vi "Release Session.vi"(8 "error in (no error)":errorcluster, 11 "Engine in":refnum<class "Engine.lvclass">) -> (0 "error out":errorcluster)   [LabVIEW 2020, in "TSnax.lvlib" / "Engine.lvclass"]
uses:
  Engine.lvclass
  Engine.lvclass/Engine.ctl
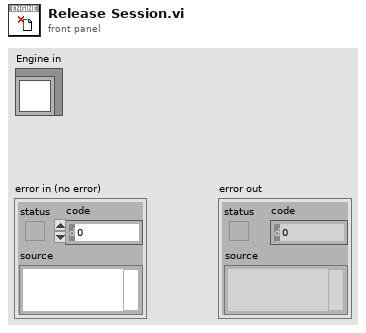
[diagram p1: front panel]
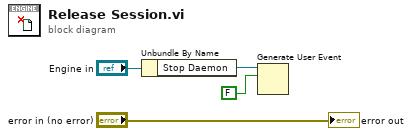
[diagram p0: block diagram]
diagram:
  n1 = Unbundle By Name("Engine in") -> ("Stop Daemon"=w2:refnum<user-event>)
  n2 = Generate User Event(user event=w2, event data cluster=FALSE ("event data")) -> ()  [unwired: 2 in, 2 out]
  "error out" <- "error in (no error)"
